vi "Post Trigger Update.vi"(8 "error in":errorcluster, 11 "Electronic Load in":refnum<class "Electronic Load.lvclass">) -> (0 "error out":errorcluster, 3 "Electronic Load out":refnum<class "Electronic Load.lvclass">)   [LabVIEW 2019, in "Electronic Load.lvlib" / "Electronic Load.lvclass"]
uses:
  Library/Electronic Load.lvclass
  Library/Electronic Load.lvclass/Electronic Load.ctl
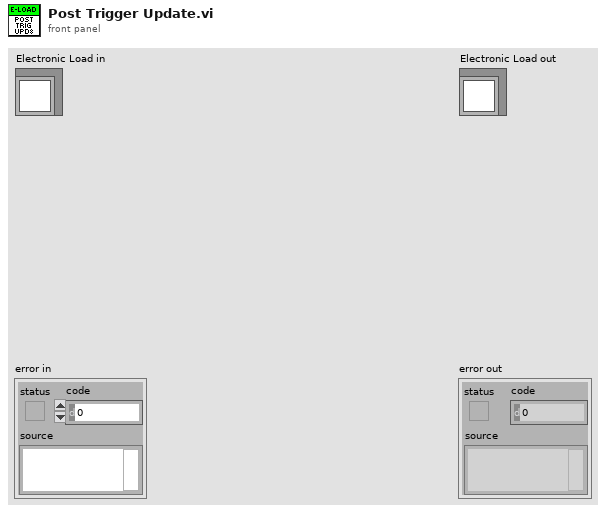
[diagram p1: front panel]
types:
  T1 = typedef "Electronic Load.lvlib/Electronic Load.lvclass/Trigger Settings.ctl" = cluster{"Mode":T2, "Initial":dbl, "Transient":dbl, "Interval":dbl, "Width":dbl, "Delay":dbl, "Data Pts":i32, "Slew Rate":dbl}
  T2 = typedef "Electronic Load.lvlib/Electronic Load.lvclass/E-Load Mode.ctl" = enum16{"Current", "Resistance", "Voltage"}
  T3 = typedef "Electronic Load.lvlib/Electronic Load.lvclass/E-Load Function.ctl" = cluster{"Mode":T2, "Input Level":dbl, "Output":bool, "Slew Rate":dbl}
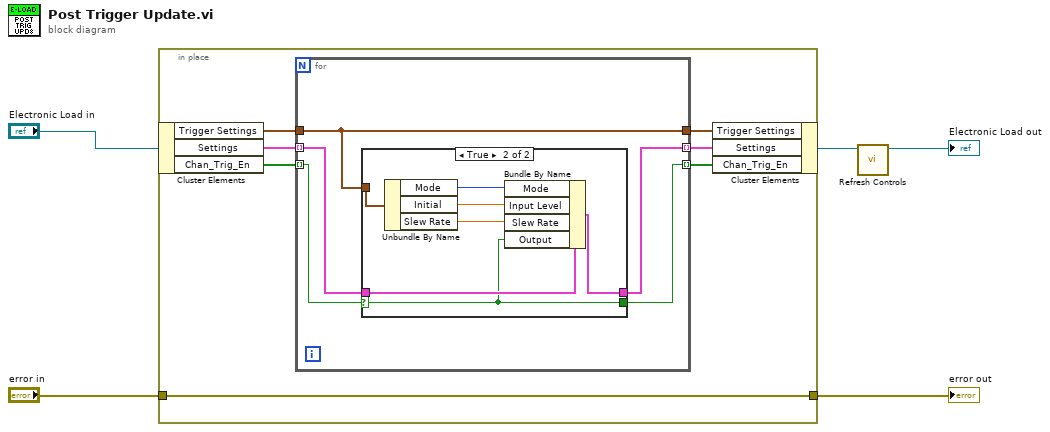
[diagram p0: block diagram]
diagram:
  n1 = in-place {
    in-place-border: "error in" -> [w12]
    in-place-border: [w12] -> w3
    n2 = in-place-cluster #1("Electronic Load in") -> ("Trigger Settings"=w11:T1, "Settings"=w10:T3[], "Chan_Trig_En"=w8:bool[])
    n3 = for {
      tunnel: w11 -> [w13]
      tunnel: w10 -> [w15] mode=indexing
      tunnel: [w13] -> w9
      tunnel: w8 -> [w17] mode=indexing
      tunnel: [w16] -> w7 mode=indexing
      tunnel: [w14] -> w6 mode=indexing
      n4 = case shown="True" w17 {
        selector: w17 -> [w18 w20]
        tunnel: [w18 w20] -> w16
        tunnel: w15 -> [w19 w26]
        tunnel: [w19 w24] -> w14
        tunnel: w13 -> [_ w25]
        frame False {
        }
        frame True {
          n5 = Unbundle By Name(w25) -> ("Mode"=w23:T2, "Initial"=w22:dbl, "Slew Rate"=w21:dbl)
          n6 = Bundle By Name(cluster=w26, "Mode"=w23, "Input Level"=w22, "Slew Rate"=w21, "Output"=w20) -> (w24:T3)
        }
      }
    }
    n7 = in-place-cluster #1("Trigger Settings"=w9, "Settings"=w6, "Chan_Trig_En"=w7) -> (w2:refnum<class "Electronic Load.lvclass">)
  }
  "error out" <- w3
  n8 = call "Refresh Controls.vi"("Electronic Load in"=w2) -> ("Electronic Load out"=→"Electronic Load out":refnum<class "Electronic Load.lvclass">)  [unwired: 9 in, 1 out]
